vi "Landfill.vi"   [LabVIEW 2014]
types:
  T1 = enum16{"Move Forward", "Move Backward", "Strafe Right", "Strafe Left"}
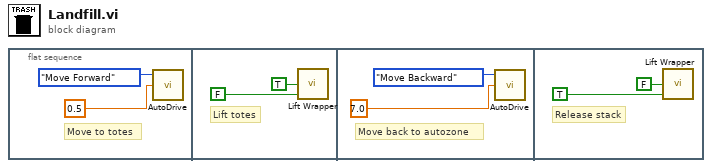
[diagram p0: block diagram]
diagram:
  n1 = flat-sequence {
    frame #0 {
      # "Move to totes"
      n2 = call "AutoDrive.vi"("Distance (ft)"=0.5 ("Feet"), "Direction"=T1."Move Forward") -> ()  [unwired: 1 in, 1 out]
    }
    frame #1 {
      # "Lift totes"
      n3 = call "Lift Wrapper.vi"("Down"=FALSE, "Up"=TRUE) -> ()  [unwired: 1 in]
    }
    frame #2 {
      # "Move back to autozone"
      n4 = call "AutoDrive.vi"("Distance (ft)"=7.0 ("Feet"), "Direction"=T1."Move Backward") -> ()  [unwired: 1 in, 1 out]
    }
    frame #3 {
      # "Release stack"
      n5 = call "Lift Wrapper.vi"("Down"=TRUE, "Up"=FALSE) -> ()  [unwired: 1 in]
    }
  }
